vi "First & Last Point.vi"(8 "Error In":errorcluster, 11 "Point Coordinates Array":i32[](array[numeric])) -> (0 "Error Out":errorcluster, 3 "First & Last Point":cluster{"X":i32, "Y":i32}[](array[cluster]))   [LabVIEW 2021, in "Image.lvlib"]
uses:
  Image.lvlib
panel:
  # "see the AlliGator License on the block diagram (Ctrl+E or Window:Show Block Diagram)"
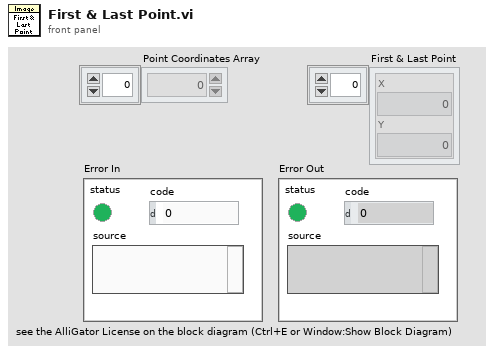
[diagram p1: front panel]
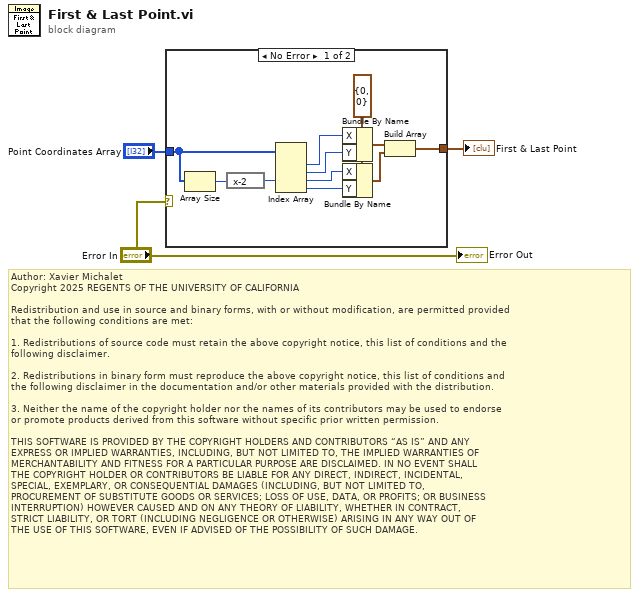
[diagram p0: block diagram]
diagram:
  # "Author: Xavier Michalet\nCopyright 2025 REGENTS OF THE UNIVERSITY OF CALIFORNIA\n\nRedistribution and use in source and binary forms, with or without modification, are permitted provided\nthat the following conditions are met:\n\n1. Redistributions of source code must retain the above copyright notice, this list of conditions and the\nfollowing disclaimer.\n\n2. Redistributions in binary form must reproduce the above copyright notice, this list of conditions and\nthe following disclaimer in the documentation and/or other materials provided with the distribution.\n\n3. Neither the name of the copyright holder nor the names of its contributors may be used to endorse \nor promote products derived from this software without specific prior written permission.\n\nTHIS SOFTWARE IS PROVIDED BY THE COPYRIGHT HOLDERS AND CONTRIBUTORS “AS IS” AND ANY \nEXPRESS OR IMPLIED WARRANTIES, INCLUDING, BUT NOT LIMITED TO, THE IMPLIED WARRANTIES OF\nMERCHANTABILITY AND FITNESS FOR A PARTICULAR PURPOSE ARE DISCLAIMED. IN NO EVENT SHALL\nTHE COPYRIGHT HOLDER OR CONTRIBUTORS BE LIABLE FOR ANY DIRECT, INDIRECT, INCIDENTAL, \nSPECIAL, EXEMPLARY, OR CONSEQUENTIAL DAMAGES (INCLUDING, BUT NOT LIMITED TO, \nPROCUREMENT OF SUBSTITUTE GOODS OR SERVICES; LOSS OF USE, DATA, OR PROFITS; OR BUSINESS\nINTERRUPTION) HOWEVER CAUSED AND ON ANY THEORY OF LIABILITY, WHETHER IN CONTRACT, \nSTRICT LIABILITY, OR TORT (INCLUDING NEGLIGENCE OR OTHERWISE) ARISING IN ANY WAY OUT OF\nTHE USE OF THIS SOFTWARE, EVEN IF ADVISED OF THE POSSIBILITY OF SUCH DAMAGE."
  n1 = case shown="No Error" "Error In" {
    tunnel: [w14 _] -> w3
    tunnel: "Point Coordinates Array" -> [w4 _]
    frame No Error {
      w9 = cluster{"X":i32, "Y":i32} {"X"=0, "Y"=0}
      n2 = Array Size(array=w4) -> (size(s)=w5:i32)
      n3 = expression code="x-2"(w5) -> (w6:i32)
      n4 = Index Array(array=w4, index #3=w6) -> (element #1=w7:i32, element #2=w8:i32, element #3=w10:i32, element #4=w11:i32)  [unwired: 3 in]
      n5 = Bundle By Name(cluster=w9, "X"=w7, "Y"=w8) -> (w12:cluster{"X":i32, "Y":i32})
      n6 = Bundle By Name(cluster=w9, "X"=w10, "Y"=w11) -> (w13:cluster{"X":i32, "Y":i32})
      n7 = Build Array(w12, w13) -> (w14:cluster{"X":i32, "Y":i32}[])
    }
    frame Error {
    }
  }
  "First & Last Point" <- w3
  "Error Out" <- "Error In"
